vi "ramsete_traject.vi"(4 "POSE TOL":dbl=0.02, 5 "B":dbl=2.0, 6 "Enabled":bool=TRUE, 7 "ZETA":dbl=0.7, 9 "TRAJ_STATE":T1, 11 "CurrentPOSE":T2) -> (0 "Err Pose":T2, 1 "AtReference":bool, 3 "CHASSIS Speeds":T5)   [LabVIEW 2019, in "PathExecution_Library.lvlib"]
uses:
  PathExecution_Library.lvlib
  CHASSIS.ctl
  TRANSLATION.ctl
  ROTATION.ctl
  POSE.ctl
  TRAJ_STATE.ctl
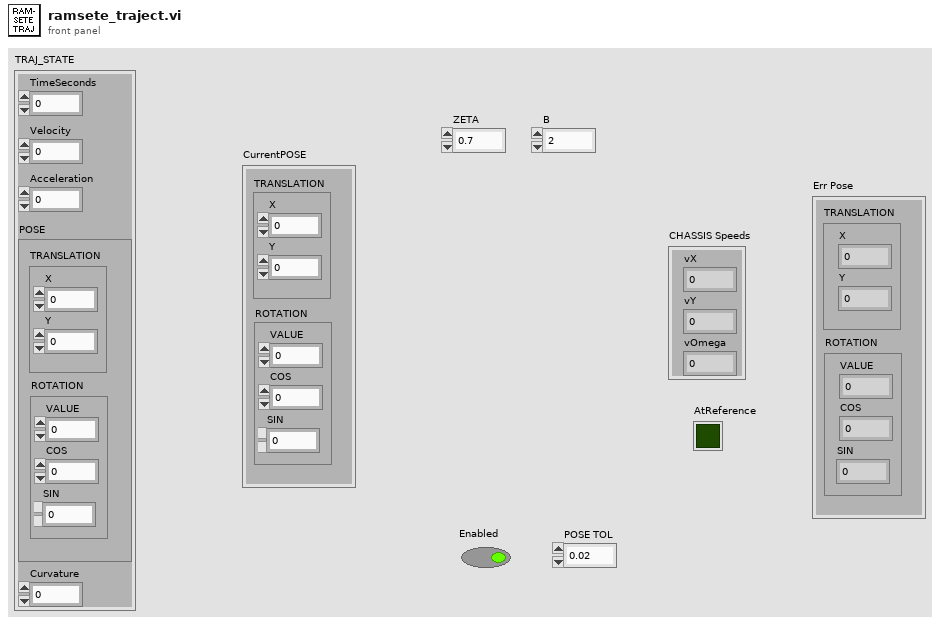
[diagram p1: front panel]
types:
  T1 = typedef "PathExecution_Library.lvlib/TRAJ_STATE.ctl" = cluster{"TimeSeconds":dbl, "Velocity":dbl, "Acceleration":dbl, "POSE":T2, "Curvature":dbl}
  T2 = typedef "PathExecution_Library.lvlib/POSE.ctl" = cluster{"TRANSLATION":T3, "ROTATION":T4}
  T3 = typedef "PathExecution_Library.lvlib/TRANSLATION.ctl" = cluster{"X":dbl, "Y":dbl}
  T4 = typedef "PathExecution_Library.lvlib/ROTATION.ctl" = cluster{"VALUE":dbl, "COS":dbl, "SIN":dbl}
  T5 = typedef "PathExecution_Library.lvlib/CHASSIS.ctl" = cluster{"vX":dbl, "vY":dbl, "vOmega":dbl}
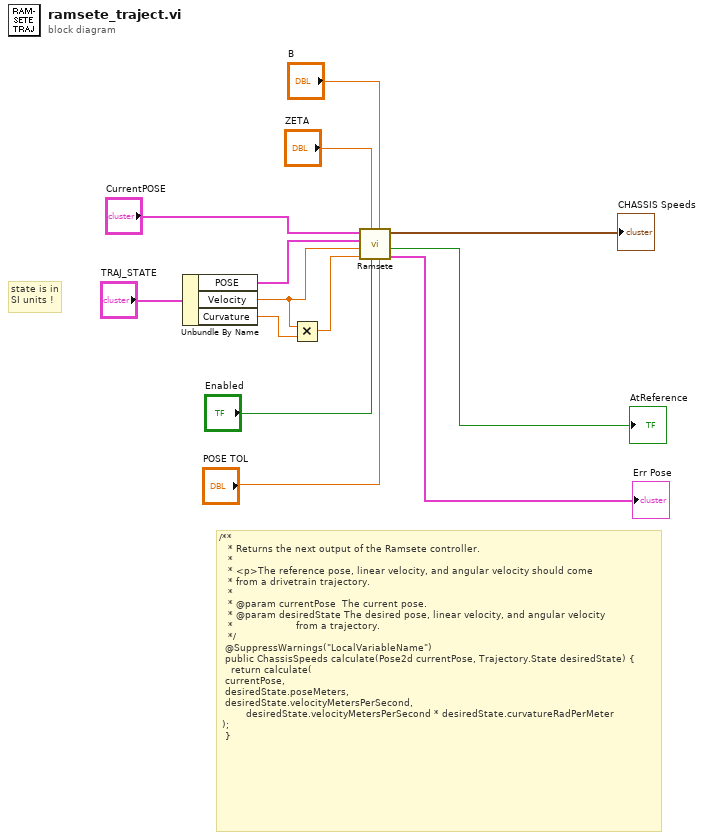
[diagram p0: block diagram]
diagram:
  # "state is in\nSI units !"
  # "/**\n   * Returns the next output of the Ramsete controller.\n   *\n   * <p>The reference pose, linear velocity, and angular velocity should come\n   * from a drivetrain trajectory.\n   *\n   * @param currentPose  The current pose.\n   * @param desiredState The desired pose, linear velocity, and angular velocity\n   *                     from a trajectory.\n   */\n  @SuppressWarnings(\"LocalVariableName\")\n  public ChassisSpeeds calculate(Pose2d currentPose, Trajectory.State desiredState) {\n    return calculate(\n\t\tcurrentPose, \n\t\tdesiredState.poseMeters, \n\t\tdesiredState.velocityMetersPerSecond,\n        \tdesiredState.velocityMetersPerSecond * desiredState.curvatureRadPerMeter\n\t);\n  }"
  n1 = Unbundle By Name("TRAJ_STATE") -> ("POSE"=w4:T2, "Velocity"=w2:dbl, "Curvature"=w3:dbl)
  n2 = Multiply(x=w2, y=w3) -> (x*y=w1:dbl)
  n3 = call "Ramsete.vi"("POSE TOL"="POSE TOL", "B"="B", "Enabled"="Enabled", "ZETA"="ZETA", "DesiredAngularVelocity"=w1, "DesiredLinearVelocity"=w2, "DesiredPOSE"=w4, "CurrentPOSE"="CurrentPOSE") -> ("Err Pose"=→"Err Pose":T2, "AtReference"=→"AtReference":bool, "CHASSIS Speeds"=→"CHASSIS Speeds":T5)  [unwired: 1 in]
